vi "ComparisionOps.vi"() -> ()   [LabVIEW 2019]
panel:
  out "x < y?":bool
  in  "a":dbl
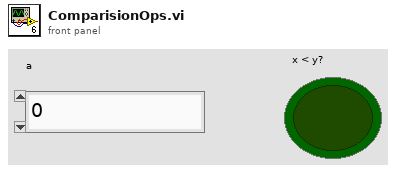
[diagram p1: front panel]
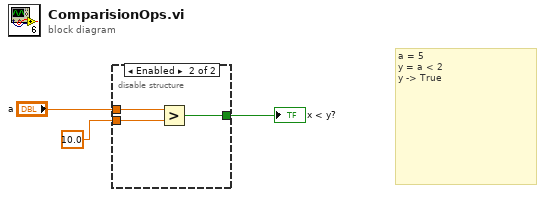
[diagram p0: block diagram]
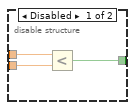
[diagram p2: hidden frame]
diagram:
  # "a = 5\ny = a < 2\ny -> True"
  n1 = disable-structure shown="Enabled" {
    disable-tunnel: "a" -> [w6 w9]
    disable-tunnel: 10.0 ("y") -> [w5 w8]
    disable-tunnel: [w4 w7] -> w1
    frame Disabled {
      n2 = Less?(x=w6, y=w5) -> (x < y?=w4:bool)
    }
    frame Enabled {
      n3 = Greater?(x=w9, y=w8) -> (0:w7:bool)
    }
  }
  "x < y?" <- w1
